vi "initialize.vi"(0 "MoAgSy_Message":refnum<class "MoAgSy_Message.lvclass">, 3 "initializationData":variant, 5 "error in (no error)":errorcluster, 7 "binaryString":string, 8 "I8 Array":i8[](array[numeric]), 9 "prependSize? (T)":bool, 11 "byteOrder (0:big-endian, network order)":T1(ring)) -> (14 "dup MoAgSy_Message":refnum<class "MoAgSy_Message.lvclass">, 17 "found?":bool, 19 "error out":errorcluster)   [LabVIEW 2009, in "MoAgSy.lvlib" / "MoAgSy_Message.lvclass"]
doc: "This is a dynamic dispatch VI to be implemented by child classes to initialize their attributes.\n\n<B>Recommendation:</B> Use Variant for initialization data."
uses:
  MoAgSy_Message.lvclass
  MoAgSy_Factory/MoAgSy_Factory.lvclass
  MoAgSy_Message.lvclass/MoAgSy_Message.ctl
  MoAgSy_AgentBase/MoAgSy_AgentBase.lvclass
panel:
  out "dup_initData":variant
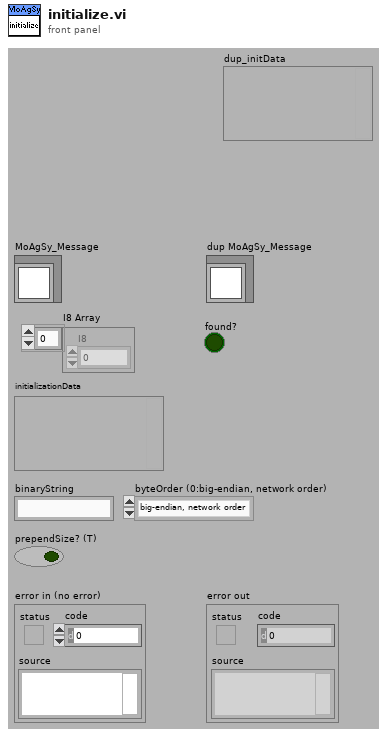
[diagram p1: front panel]
types:
  T1 = enum16{"big-endian, network order", "native, host order", "little-endian"}
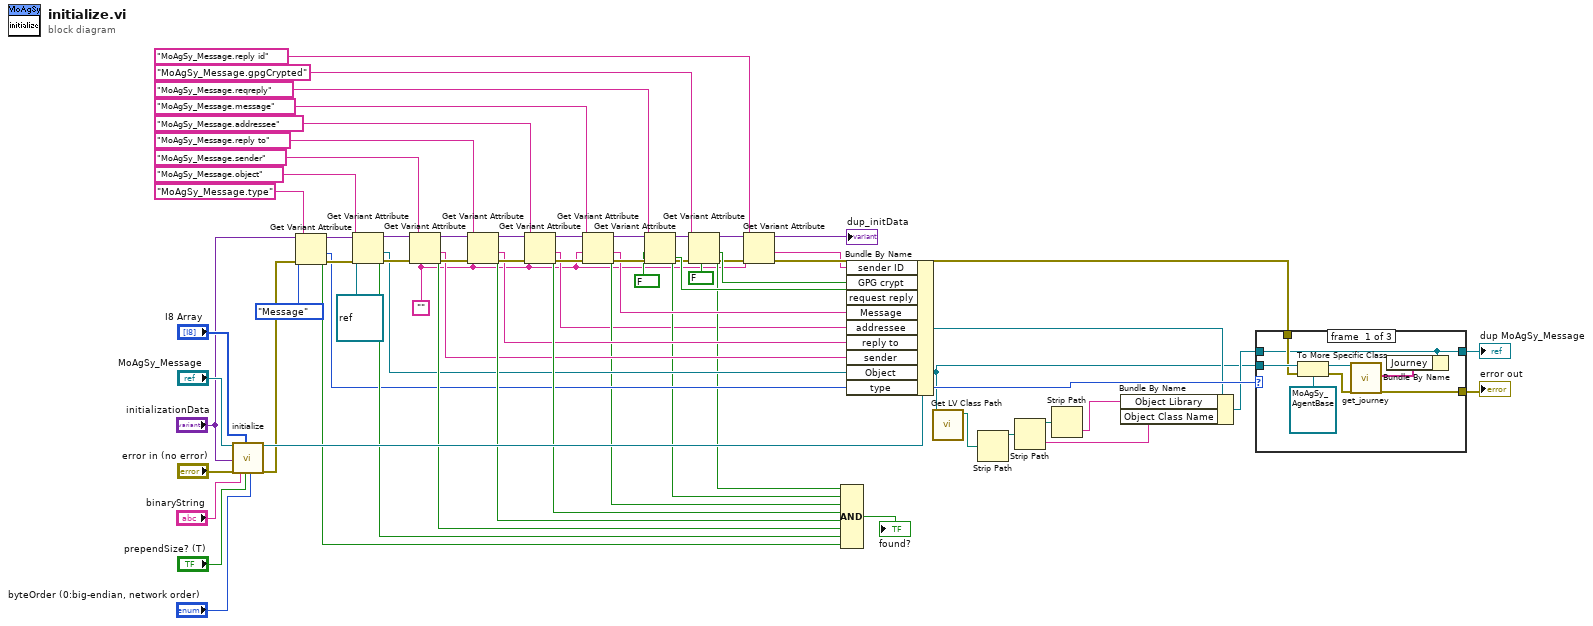
[diagram p0: block diagram]
diagram:
  w3 = "" ("addressee")
  n1 = call-parent "initialize.vi"("HGF_Factory"="MoAgSy_Message", "initializationData"="initializationData", "error in (no error)"="error in (no error)", "binaryString"="binaryString", "I8 Array"="I8 Array", "prependSize? (T)"="prependSize? (T)", "byteOrder (0:big-endian, network order)"="byteOrder (0:big-endian, network order)") -> ("dup HGF_Factory"=w62:refnum<class "MoAgSy_Message.lvclass">, "error out"=w41:errorcluster)  [unwired: 11 out]
  n2 = Get Variant Attribute(Variant="initializationData", name="MoAgSy_Message.type", default value (empty Variant)=enum16{"mobile Agent", "Visitor", "Message"}."Message" ("type"), error in=w41) -> (duplicate Variant=w53:variant, found=w42:bool, value=w38:enum16{"mobile Agent", "Visitor", "Message"}, error out=w52:errorcluster)
  n3 = Get Variant Attribute(Variant=w53, name="MoAgSy_Message.object", default value (empty Variant)=refnum<class> refnum ("Object"), error in=w52) -> (duplicate Variant=w57:variant, found=w43:bool, value=w29:refnum<class>, error out=w56:errorcluster)
  n4 = Get Variant Attribute(Variant=w57, name="MoAgSy_Message.sender", default value (empty Variant)=w3, error in=w56) -> (duplicate Variant=w60:variant, found=w44:bool, value=w39:string, error out=w59:errorcluster)
  n5 = Get Variant Attribute(Variant=w60, name="MoAgSy_Message.reply to", default value (empty Variant)=w3, error in=w59) -> (duplicate Variant=w50:variant, found=w45:bool, value=w40:string, error out=w48:errorcluster)
  n6 = Get Variant Attribute(Variant=w50, name="MoAgSy_Message.addressee", default value (empty Variant)=w3, error in=w48) -> (duplicate Variant=w24:variant, found=w46:bool, value=w8:string, error out=w25:errorcluster)
  n7 = Get Variant Attribute(Variant=w24, name="MoAgSy_Message.message", default value (empty Variant)=w3, error in=w25) -> (duplicate Variant=w22:variant, found=w23:bool, value=w17:string, error out=w21:errorcluster)
  n8 = Get Variant Attribute(Variant=w22, name="MoAgSy_Message.reqreply", default value (empty Variant)=FALSE, error in=w21) -> (duplicate Variant=w14:variant, found=w15:bool, value=w18:bool, error out=w13:errorcluster)
  n9 = Get Variant Attribute(Variant=w14, name="MoAgSy_Message.gpgCrypted", default value (empty Variant)=FALSE, error in=w13) -> (duplicate Variant=w6:variant, found=w10:bool, value=w9:bool, error out=w7:errorcluster)
  n10 = Get Variant Attribute(Variant=w6, name="MoAgSy_Message.reply id", default value (empty Variant)=w3, error in=w7) -> (duplicate Variant=→"dup_initData":variant, value=w2:string, error out=w4:errorcluster)  [unwired: 1 out]
  n11 = Compound Arithmetic op=AND(w10, w15, w23, w46, w45, w44, w43, w42) -> (→"found?":bool)
  n12 = Bundle By Name(cluster=w62, "sender ID"=w2, "GPG crypt"=w9, "request reply"=w18, "Message"=w17, "addressee"=w8, "reply to"=w40, "sender"=w39, "Object"=w29, "type"=w38) -> (w31:refnum<class "MoAgSy_Message.lvclass">)
  n13 = call <vilib>:"Get LV Class Path.vi"("object"=w29) -> ("class path"=w32:path)  [unwired: 1 in, 9 out]
  n14 = Strip Path(path=w32) -> (stripped path=w33:path)  [unwired: 1 out]
  n15 = Strip Path(path=w33) -> (stripped path=w35:path, name=w34:string)
  n16 = Strip Path(path=w35) -> (name=w36:string)  [unwired: 1 out]
  n17 = Bundle By Name(cluster=w31, "Object Library"=w36, "Object Class Name"=w34) -> (w30:refnum<class "MoAgSy_Message.lvclass">)
  n18 = case shown="\"mobile Agent\"" w38 {
    tunnel: w30 -> [w70 w78 w80]
    tunnel: w29 -> [w76 _ _]
    tunnel: [w70 w78 w80] -> w37
    tunnel: w4 -> [w71 w77 w79]
    tunnel: [w69 w77 w79] -> w27
    frame #0 {
      n19 = To More Specific Class(target class=refnum<class "MoAgSy_AgentBase.lvclass"> refnum ("HGF_AgentBaseClasses.lvlib:HGF_Agent.lvclass"), reference=w76, error in=w71) -> (specific class reference=w74:refnum<class "MoAgSy_AgentBase.lvclass">, error out=w73:errorcluster)
      n20 = call "get_journey.vi"("HGF_Agent in"=w74, "error in (no error)"=w73) -> ("journey"=w72:string[], "error out"=w69:errorcluster)  [unwired: 16 out]
      n21 = Bundle By Name(cluster=w70, "Journey"=w72) -> ()  [unwired: 1 out]
    }
    frame #1 {
    }
    frame #2 {
    }
  }
  "error out" <- w27
  "dup MoAgSy_Message" <- w37
